vi "Get Channel Blocks.vi"(11 "Transfer Configuration in":refnum<class "Transfer Configuration.lvclass">) -> (2 "channel blocks":T1[](array[typedef]) {"buffer offset" format="%d bytes"}, 3 "Transfer Configuration out":refnum<class "Transfer Configuration.lvclass">)   [LabVIEW 2017, in "DSF Core.lvlib" / "Transfer Configuration.lvclass"]
uses:
  Transfer Configuration.lvclass
  Typedefs/DSF Runtime Channel Block.ctl
  DSF Configuration API/Public/Controls/DSF Data Type.ctl
  Transfer Configuration.lvclass/Transfer Configuration.ctl
  DSF Core.lvlib
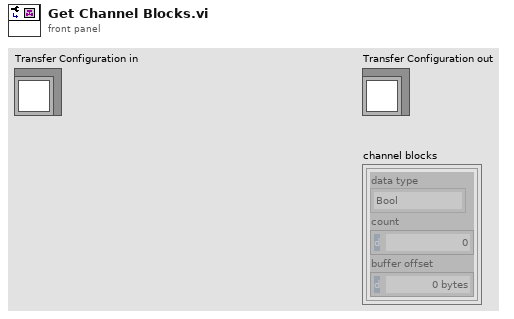
[diagram p1: front panel]
types:
  T1 = typedef "DSF Core.lvlib/DSF Runtime Channel Block.ctl" = cluster{"data type":T2, "count":u64, "buffer offset":u64}
  T2 = typedef "DSF Core.lvlib/DSF Data Type.ctl" = enum8{"Bool", "SGL", "DBL", "I8", "I16", "I32", "I64", "U8", "U16", "U32", "U64"}
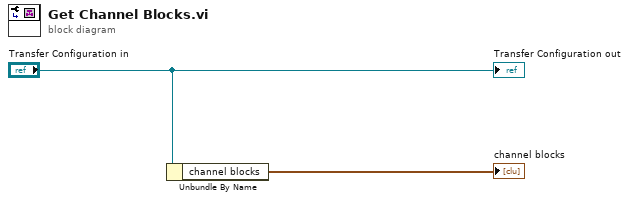
[diagram p0: block diagram]
diagram:
  n1 = Unbundle By Name("Transfer Configuration in") -> ("channel blocks"=→"channel blocks":T1[])
  "Transfer Configuration out" <- "Transfer Configuration in"
